vi "Init.vi"(8 "error in (no error)":errorcluster, 10 "Active Sequence File":refnum<k7>, 11 "Engine In":refnum<k7>) -> (0 "error out":errorcluster, 2 "Engine Out":refnum<k7>, 3 "Sequence Call Step  Dictionary out":refnum<class "Sequence Call Step Dictionary.lvclass">)   [LabVIEW 2018, in "Sequence Call Step Dictionary.lvlib" / "Sequence Call Step Dictionary.lvclass"]
uses:
  Sequence Call Step Dictionary.lvclass
  Sequence Call Step Dictionary.lvclass/Sequence Call Step Dictionary.ctl
  Controls/Sequence Call Step.ctl
  Controls/Parameter.ctl
  Private Methods/Read Database.vi
  Private Methods/Write Database.vi
  Plugins/TestStand API Tools (TSAT).lvlibp/Sequence File Actions/TSAT Sequence File Actions.lvlib
  Plugins/TestStand API Tools (TSAT).lvlibp/Sequence Actions/TSAT Sequence Actions.lvlib
  Plugins/TestStand API Tools (TSAT).lvlibp/TSAT Utilities/TSAT Utilities.lvlib
  Plugins/TestStand API Tools (TSAT).lvlibp/Step Actions/TSAT Step Actions.lvlib
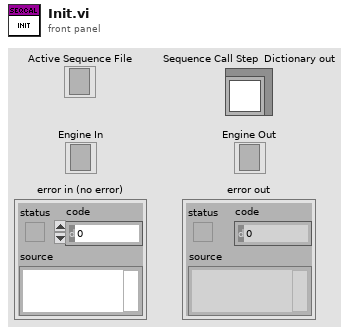
[diagram p1: front panel]
types:
  T1 = typedef "Sequence Call Step Dictionary.lvlib/Sequence Call Step Dictionary.lvclass/Parameter.ctl" = cluster{"Name":string, "PropertyObject Type":enum16{"Container", "String", "Boolean", "Number", "NamedType", "Reference", "Array", "Aperture Time"}}
  T2 = typedef "Sequence Call Step Dictionary.lvlib/Sequence Call Step Dictionary.lvclass/Sequence Call Step.ctl" = cluster{"Sequence Call Step Reference":refnum<k7>, "Sequence Call Parameters":T1[]}
  T3 = enum16{"Container", "String", "Boolean", "Number", "NamedType", "Reference", "Array", "Aperture Time"}
  T4 = enum16{"Container", "String", "Boolean", "Number", "NamedType", "Reference", "Array"}
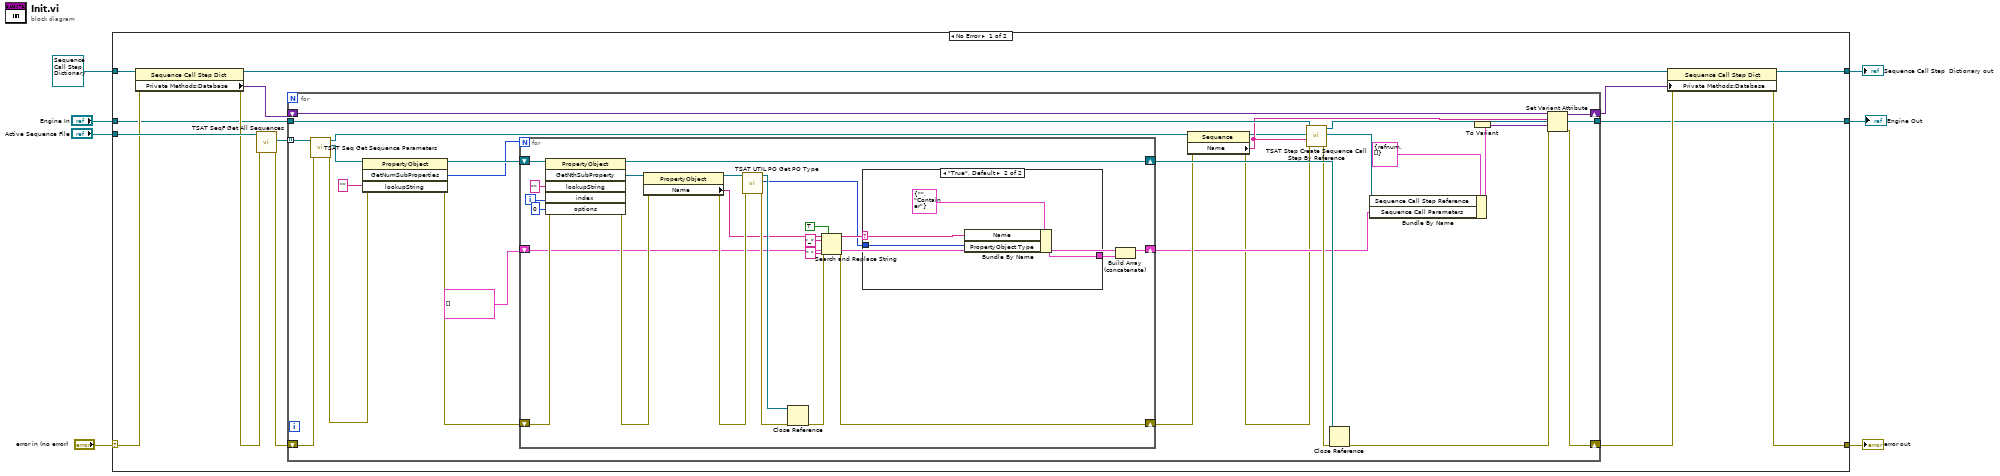
[diagram p0: block diagram]
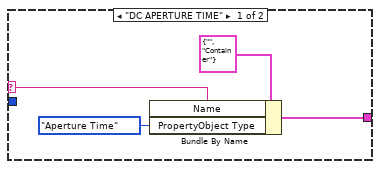
[diagram p2: hidden frame]
diagram:
  n1 = case shown="No Error" "error in (no error)" {
    selector: "error in (no error)" -> [w20 w82]
    tunnel: [w11 w82] -> w6
    tunnel: [w9 w81] -> w4
    tunnel: refnum<class "Sequence Call Step Dictionary.lvclass"> refnum ("Sequence Call Step  Dictionary in") -> [w16 w81]
    tunnel: "Active Sequence File" -> [w21 _]
    tunnel: "Engine In" -> [w14 w80]
    tunnel: [w13 w80] -> w1
    frame No Error {
      n2 = property class="Sequence Call Step Dict"(reference=w16, error in=w20) -> (reference out=w10:refnum<class "Sequence Call Step Dictionary.lvclass">, error out=w17:errorcluster, "Private Methods:Database"=w12:variant)
      n3 = call "TSAT SeqF Get All Sequences.vi"("Error In"=w17, "Sequence File In"=w21) -> ("Error Out"=w19:errorcluster, "Array Of Sequences"=w18:refnum<k7>[])  [unwired: 7 in, 1 out]
      n4 = for {
        shift-right: [w30] -> w15
        shift-left: w19 -> [w47]
        tunnel: w18 -> [w48] mode=indexing
        tunnel: w14 -> [w36]
        tunnel: [w35] -> w13
        shift-right: [w29] -> w8
        shift-left: w12 -> [w28]
        n5 = call "TSAT Seq Get Sequence Parameters.vi"("Error in"=w47, "Sequence Reference In"=w48) -> ("Error out"=w40:errorcluster, "Parameters"=w41:refnum<k7>, "Sequence Reference Out"=w38:refnum<k7>)  [unwired: 7 in]
        n6 = invoke class="PropertyObject" method="GetNumSubProperties"(reference=w41, error in=w40, "lookupString"="") -> (reference out=w44:refnum<k7>, error out=w45:errorcluster, "GetNumSubProperties"=w42:i32)  [unwired: 1 in, 1 out]
        n7 = for {
          N: w42 -> [_]
          shift-right: [w56] -> w37
          shift-left: w45 -> [w71]
          shift-right: [w69] -> w43
          shift-left: w44 -> [w70]
          shift-right: [w50] -> w25
          shift-left: T1[] [] -> [w49]
          i -> [w67]
          n8 = invoke class="PropertyObject" method="GetNthSubProperty"(reference=w70, error in=w71, "lookupString"="", "index"=w67, "options"=0) -> (reference out=w69:refnum<k7>, error out=w64:errorcluster, "GetNthSubProperty"=w65:refnum<k7>)  [unwired: 1 in, 3 out]
          n9 = property class="PropertyObject"(reference=w65, error in=w64) -> (reference out=w61:refnum<k7>, error out=w63:errorcluster, "Name"=w59:string)
          n10 = call "TSAT UTIL PO Get PO Type.vi"("error in (no error)"=w63, "PropertyObject In"=w61) -> ("error out"=w62:errorcluster, "PropertyObject Type"=w52:T4, "PropertyObject Out"=w60:refnum<k7>)  [unwired: 7 in]
          n11 = Close Reference(reference=w60, error in (no error)=w62) -> (error out=w57:errorcluster)
          n12 = Search and Replace String(replace all?=TRUE ("replace all? (F)"), input string=w59, search string="_", replace string=" " ("replace string (\"\")"), error in=w57) -> (result string=w53:string, error out=w56:errorcluster)  [unwired: 3 in, 2 out]
          n13 = case shown="\"True\", Default" w53 {
            selector: w53 -> [w75 w78]
            tunnel: w52 -> [_ w77]
            tunnel: [w74 w79] -> w51
            frame "DC APERTURE TIME" {
              n14 = Bundle By Name(cluster=T1 {"Name"="", "PropertyObject Type"=enum."Container"} ("output cluster"), "Name"=w75, "PropertyObject Type"=T3."Aperture Time") -> (w74:T1)
            }
            frame "True", Default {
              n15 = Bundle By Name(cluster=T1 {"Name"="", "PropertyObject Type"=enum."Container"} ("output cluster"), "Name"=w78, "PropertyObject Type"=w77) -> (w79:T1)
            }
          }
          n16 = Build Array (concatenate)(w49, w51) -> (w50:T1[])
        }
        n17 = property class="Sequence"(reference=w38, error in=w37) -> (reference out=w22:refnum<k7>, error out=w23:errorcluster, "Name"=w24:string)
        n18 = call "TSAT Step Create Sequence Call Step By Reference.vi"("Error In"=w23, "Step Name"=w24, "Sequence to Call"=w22, "Engine In"=w36) -> ("Error Out"=w39:errorcluster, "Step Reference"=w34:refnum<k7>, "Engine Out"=w35:refnum<k7>)  [unwired: 5 in]
        n19 = Close Reference(reference=w43, error in (no error)=w39) -> (error out=w31:errorcluster)
        n20 = Bundle By Name(cluster=T2 {"Sequence Call Step Reference"=refnum, "Sequence Call Parameters"=[]} ("Cluster"), "Sequence Call Step Reference"=w34, "Sequence Call Parameters"=w25) -> (w33:T2)
        n21 = To Variant(anything=w33) -> (Variant=w32:variant)
        n22 = Set Variant Attribute(Variant=w28, name=w24, value=w32, error in=w31) -> (Variant out=w29:variant, error out=w30:errorcluster)  [unwired: 1 out]
      }
      n23 = property class="Sequence Call Step Dict"(reference=w10, error in=w15, "Private Methods:Database"=w8) -> (reference out=w9:refnum<class "Sequence Call Step Dictionary.lvclass">, error out=w11:errorcluster)
    }
    frame Error {
    }
  }
  "error out" <- w6
  "Sequence Call Step  Dictionary out" <- w4
  "Engine Out" <- w1
